vi "Test Test Case Title Correct When Collecting Method Result.vi"(8 "error in (no error)":errorcluster, 11 "Test Case In":refnum<class "Result Collector Tests.lvclass">) -> (0 "error out":errorcluster, 3 "Test Case Out":refnum<class "Result Collector Tests.lvclass">)   [LabVIEW 2020, in "Result Collector Tests.lvclass"]
uses:
  Result Collector Tests.lvclass
  C:/Program Files (x86)/National Instruments/LabVIEW 2020/vi.lib/Astemes/LUnit/Test Case.lvclass
  source/Framework/Result Collector/Result Collector.lvclass
  source/Rewrite Project/Result/Result.ctl
  source/Rewrite Project/Result/Status.ctl
  source/Rewrite Project/Result/Type.ctl
  source/Framework/Result Collector/Result Collector.lvclass/Result Collector.ctl
  <vilib>/Astemes/LUnit/Test Case.lvclass/Test Case.ctl
  7d523b10-b8d1-4baa-9334-5865d033fd32.vi
  source/Framework/Result Collector/Public/API/Collect Method Results.vi
  <vilib>/AdvancedString/Delimited String to 1D String Array.vi
  <vilib>/AdvancedString/1D String Array to Delimited String.vi
  source/Framework/Result Collector/Public/API/Collect Case Result.vi
  source/Framework/Result Collector/Public/API/Collect Suite Result.vi
  <vilib>/Astemes/LUnit/Palette/Pass.vi
  <vilib>/Astemes/LUnit/Palette/Fail.vi
  <vilib>/Astemes/LUnit/Compare Variants.vi
  <vilib>/Astemes/LUnit/Describe Comparison.vi
  <vilib>/Astemes/LUnit/Set Assertion Type.vi
  <vilib>/Astemes/LUnit/Add test result.vi
  <vilib>/Astemes/LUnit/Variant to string.vi
  <vilib>/Astemes/LUnit/LUnit Record Assertion Result.vi
  <vilib>/Astemes/LUnit/LUnit Aggregate Assertion Results.vi
  <vilib>/Astemes/LUnit/Method Result/LUnit Merge Status.vi
  <vilib>/Astemes/LUnit/LUnit Concatenate result strings.vi
  <vilib>/Utility/Data Type/Get Type Information.vi
  <vilib>/Utility/LVClass/Get LV Class Name.vi
  source/Rewrite Project/Result/Result.lvlib
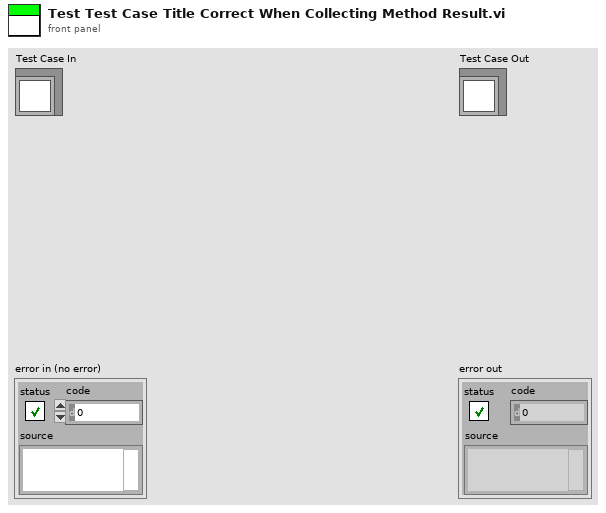
[diagram p1: front panel]
types:
  T1 = typedef "Result.lvlib/Result.ctl" = cluster{"Name":string, "Message":string, "Description":string, "Status":T2, "Result Type":T3, "Execution Time":dbl}
  T2 = typedef "Result.lvlib/Status.ctl" = enum16{"", "Passed", "Failed", "Error", "Skipped", "Setup Error", "Broken", "Teardown Error"}
  T3 = typedef "Result.lvlib/Type.ctl" = enum16{"Method", "Case", "Suite", "Pass", "Fail", "Skip", "Pass if", "Fail if", "Pass if Error", "Fail if Error", "Pass if Equal", "Fail if Equal"}
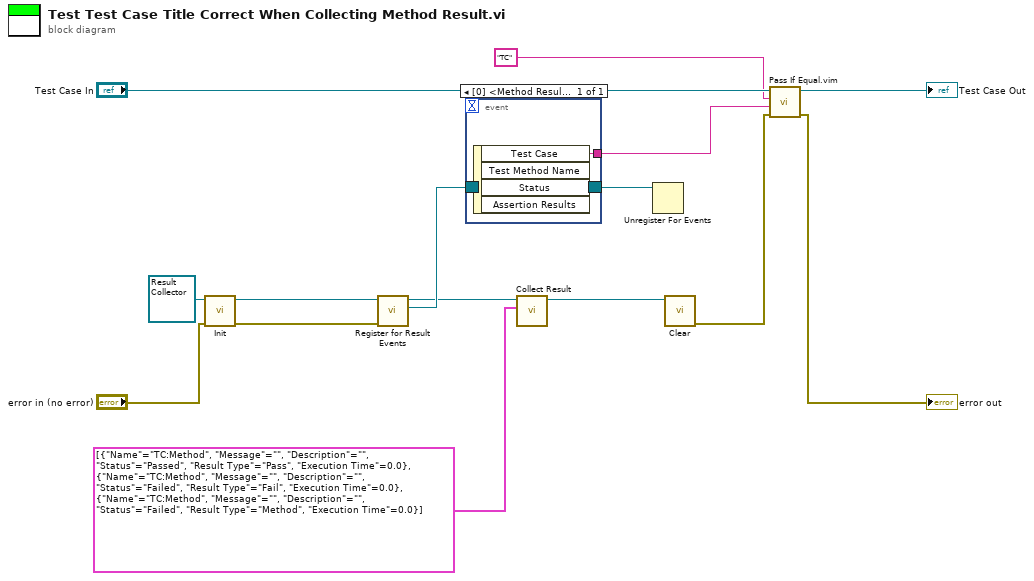
[diagram p0: block diagram]
diagram:
  n1 = call-dynamic "Init.vi"("error in (no error)"="error in (no error)", "Report Generator In"=refnum<class "Result Collector.lvclass"> refnum) -> ("error out"=w11:errorcluster, "Report Generator Out"=w12:refnum<class "Result Collector.lvclass">)  [unwired: 8 in]
  n2 = call "Register for Result Events.vi"("error in (no error)"=w11, "Result Collector In"=w12) -> ("Event Registration Refnum"=w9:refnum<event-registration>, "Result Collector Out"=w7:refnum<class "Result Collector.lvclass">)  [unwired: 7 in, 1 out]
  n3 = event shown="[0] <Method Results>: User Event" {
    selector: w9 -> [_]
    dyn-events: [_] -> w8
    timeout: _ -> [_]
    tunnel: [w16] -> w4
    event User Event {
      n4 = event-data() -> ("Test Case"=w16:string)  [unwired: 1 in, 3 out]
    }
  }
  n5 = call "Collect Result.vi"("Results"=T1[] [{"Name"="TC:Method", "Message"="", "Description"="", "Status"=enum."Passed", "Result Type"=enum."Pass", "Execution Time"=0.0}, {"Name"="TC:Method", "Message"="", "Description"="", "Status"=enum."Failed", "Result Type"=enum."Fail", "Execution Time"=0.0}, {"Name"="TC:Method", "Message"="", "Description"="", "Status"=enum."Failed", "Result Type"=enum."Method", "Execution Time"=0.0}], "Report Generator In"=w7) -> ("Report Generator Out"=w6:refnum<class "Result Collector.lvclass">)  [unwired: 9 in]
  n6 = Unregister For Events(event registration refnum=w8) -> ()  [unwired: 1 in, 1 out]
  n7 = call-dynamic "Clear.vi"("Report Generator In"=w6) -> ("error out"=w2:errorcluster)  [unwired: 9 in, 1 out]
  n8 = call "Pass If Equal.vim"("error in (no error)"=w2, "Actual"=w4, "Expected"="TC" ("Case"), "LUnit Test Case In"="Test Case In") -> ("error out"=→"error out":errorcluster, "LUnit Test Case Out"=→"Test Case Out":refnum<class "Result Collector Tests.lvclass">)  [unwired: 6 in]
